vi "MeasurePWM.vi"(11 "FPGA I/O In":refnum<k21>="sbRIO-9651 Socket\\PMOD_I2C_SCL1_in") -> ()   [LabVIEW 2019]
uses:
  TypeDefs/TimeSymbol.ctl
  <vilib>/Platform/TimedLoop/XDataNode/timing_clust.ctl
  <vilib>/Platform/TimedLoop/XDataNode/nitl_modes.ctl
  <vilib>/Platform/TimedLoop/XDataNode/wakeup.ctl
  <vilib>/rvi/Emulation/niFpgaSctlEmulationGetInTimedLoop.vi
  <vilib>/rvi/Emulation/niFpgaEmulationReportErrorSimple.vi
  <vilib>/rvi/Emulation/niFpgaGetClockAttributes.vi
  <vilib>/rvi/Emulation/niFpgaCriticalErrorInLSC.vi
  <vilib>/rvi/eio/common/nirviEmuTemplateMethod_errors.vi
  <instrlib>/_niInstr/Basic Elements/v1/FPGA/Private/D Latch U32.vi
  <vilib>/platform/TimedLoop/XDataNode/XDataNode.xnode
  <vilib>/eio/EIONode/EIONode.xnode
  <instrlib>/_niInstr/Basic Elements/v1/FPGA/niInstr Basic Elements v1 FPGA.lvlib
  <vilib>/Platform/TimedLoop/XDataNode/XDNodeRunTimeDep.lvlib
panel:
  out "s? t:f":T1=enum."Marker"
  out "Valid":bool
  in  "signal":bool
  out "TotalTime":u32
  out "OffTime":u32
  out "OnTime":u32
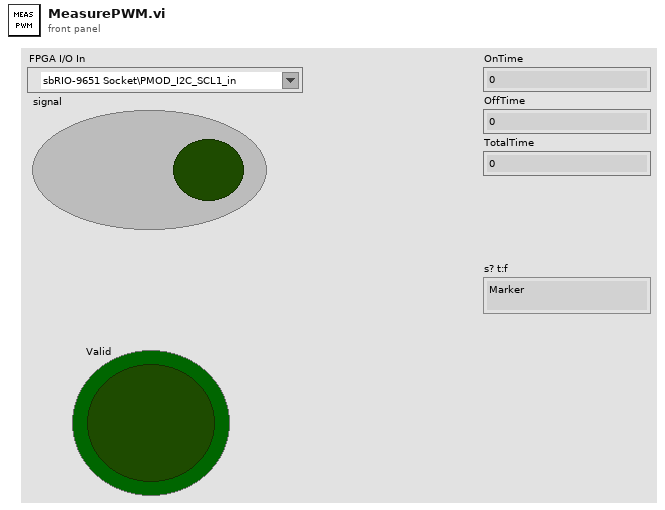
[diagram p1: front panel]
types:
  T1 = typedef "TimeSymbol.ctl" = enum16{"0", "1", "Marker", "Invalid"}
  T2 = typedef "XDNodeRunTimeDep.lvlib/timing_clust.ctl" = cluster{"Expected End [f-1]":u64, "Actual End [f-1]":u64, "Finished Late? [f-1]":bool, "Expected End [i-1]":u64, "Actual End [i-1]":u64, "Finished Late? [i-1]":bool, "Expected Start [i]":u64, "Actual Start [i]":u64, "Expected Start [f]":u64, "Actual Start [f]":u64, "Source Name":string, "Structure Name":string, "Period":i64, "Deadline":i64, "Offset":i64, "Start":i64, "Priority":i32, "Timeout":i32, "Mode":T3, "Wakeup Reason":T4, "Error":errorcluster, "Source Type":string, "Secondary Source Type":string, "Global End Time":u64, "Global Start Time":u64, "Frame Duration":u64, "Iteration Duration":u64, "Assigned CPU":i32, "I/O Scan Engine Mode":u32}
  T3 = typedef "XDNodeRunTimeDep.lvlib/nitl_modes.ctl" = enum32{"No Change", "Process missed periods, maintain original phase", "Discard missed periods, maintain original phase", "Process missed periods, ignore original phase", "Discard missed periods, ignore original phase"}
  T4 = typedef "XDNodeRunTimeDep.lvlib/wakeup.ctl" = enum32{"Normal", "Aborted", "Asynchronous wakeup", "Timing source error", "Timed loop error", "Timeout"}
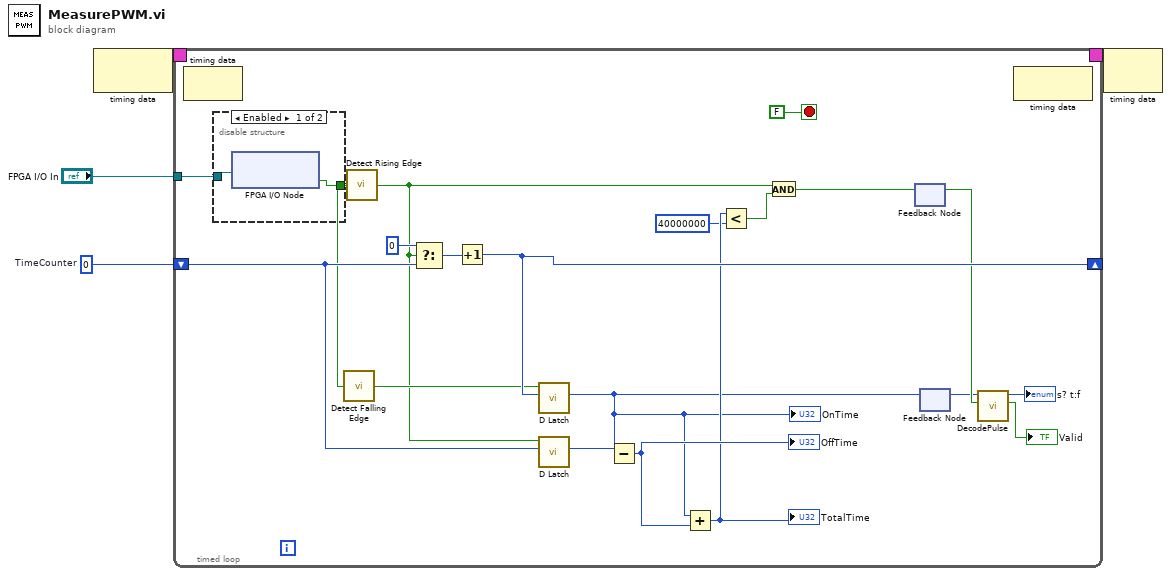
[diagram p0: block diagram]
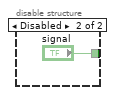
[diagram p2: hidden frame]
diagram:
  w4 = u32 0  # TimeCounter
  n1 = node-c288() -> (w3:T2)  [unwired: 1 in]
  n2 = timed-loop {
    tunnel: "FPGA I/O In" -> [w24]
    shift-right: [w21] -> _
    shift-left: w4 -> [w19]
    timing: w3 -> [_]
    timing-out: [_] -> w2
    stop <- FALSE stop-if-true
    n3 = node-c288() -> ()  [unwired: 1 in, 1 out]
    n4 = disable-structure shown="Enabled" {
      disable-tunnel: w24 -> [w28 _]
      disable-tunnel: [w27 "signal"] -> w17
      frame Enabled {
        n5 = xnode "FPGA I/O Node"("FPGA I/O In"=w28) -> ("I/O Item"=w27:bool)  [unwired: 1 out]
      }
      frame Disabled {
      }
    }
    n6 = call <instrlib>:"Detect Falling Edge.vi"("signal"=w17) -> ("edge detected"=w18:bool)  [unwired: 14 in]
    n7 = call <instrlib>:"Detect Rising Edge.vi"("signal"=w17) -> ("edge detected"=w14:bool)  [unwired: 14 in]
    n8 = Select(t=u32 0, s=w14, f=w19) -> (s? t:f=w23:u32)
    n9 = Increment(x=w23) -> (x+1=w21:u32)
    n10 = call-poly <instrlib>:"D Latch.vi"("d"=w21, "s"=w18) -> ("q"=w10:u32)  [unwired: 9 in]
    "OnTime" <- w10
    n11 = call-poly <instrlib>:"D Latch.vi"("d"=w19, "s"=w14) -> ("q"=w16:u32)  [unwired: 9 in]
    n12 = Subtract(x=w16, y=w10) -> (x-y=w15:u32)
    "OffTime" <- w15
    n13 = Add(x=w10, y=w15) -> (x+y=w13:u32)
    "TotalTime" <- w13
    n14 = Less?(x=w13, y=u32 40000000) -> (x < y?=w11:bool)
    n15 = And(x=w14, y=w11) -> (x .and. y?=w9:bool)
    n16 = feedback-in #1(w9) -> ()
    n17 = feedback #1() -> (w6:bool)  [unwired: 1 in]
    n18 = feedback-in #2(w10) -> ()
    n19 = feedback #2() -> (w5:u32)  [unwired: 1 in]
    n20 = call "DecodePulse.vi"("ValidInput"=w6, "OnTime"=w5) -> ("OutputValid"=→"Valid":bool, "s? t:f"=→"s? t:f":T1)  [unwired: 8 in]
    n21 = node-c288() -> ()  [unwired: 1 in, 1 out]
  }
  n22 = node-c288(w2) -> ()  [unwired: 1 out]
